vi "presentation_software.vi"() -> ()   [LabVIEW 2014]
uses:
  stateCtl.ctl
  <vilib>/Instr/_visa.llb/VISA Configure Serial Port (Instr).vi
panel:
  in  "AnalogOutputDT":dbl(slide) scale=0.0..100.0
  out "Led1":bool
  in  "Output1":bool
  out "Led0":bool
  in  "Output0":bool
  out "S6":dbl
  out "S5":dbl
  out "S4":dbl
  out "S3":dbl
  out "S2":dbl
  out "S1":dbl
  out "S0":dbl
  in  "Tab Control":T1(tab)
  out "Frequency":dbl(graph)
  out "Temperature 1":dbl(graph)
  out "Temperature 2":dbl(graph)
  out "Load Cell 1":dbl(graph)
  out "Load Cell 2":dbl(graph)
  out "Vibration":dbl(graph)
  out "Analog Output":dbl(graph)
  out "exitLed":bool
  out "statusBar":string="     "
  in  "startButton":bool
  out "stopLed":bool
  out "startLed":bool
  in  "VISA Serial Port":refnum<visa-resource-name>
  in  "exitButton":bool
  in  "stopButton":bool
  out "FE":string
  out "FP":string
  out "isRunning":bool
  out "state":T2=enum."exit"
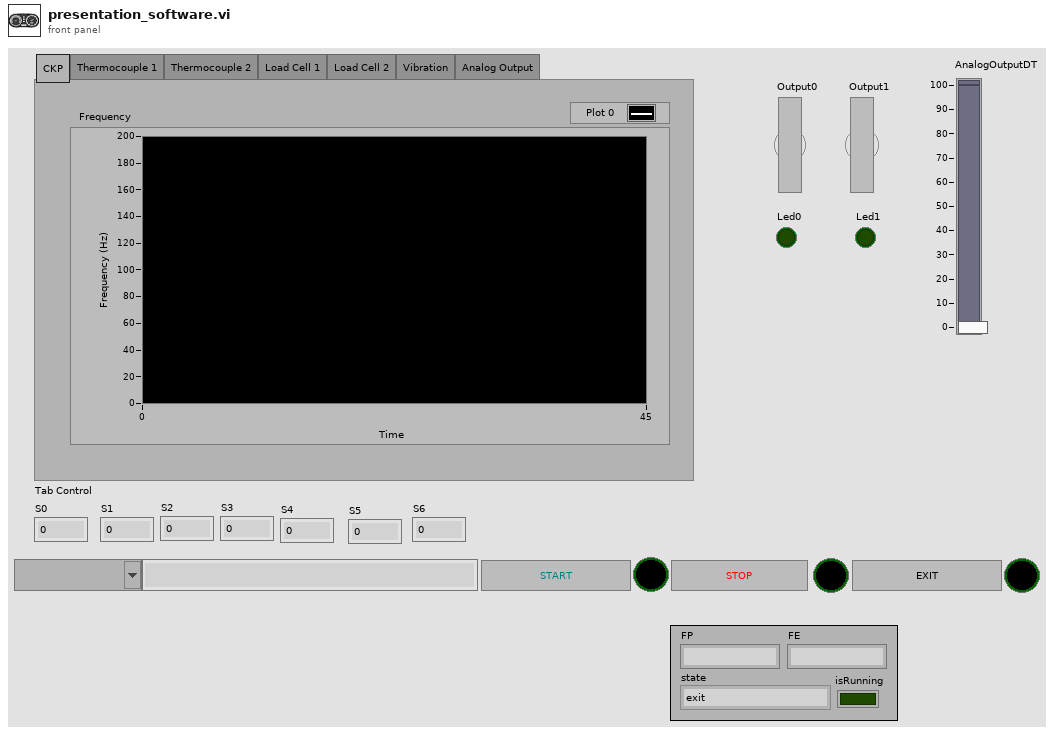
[diagram p1: front panel]
types:
  T1 = enum32{"CKP", "Thermocouple 1", "Thermocouple 2", "Load Cell 1", "Load Cell 2", "Vibration", "Analog Output"}
  T2 = typedef "stateCtl.ctl" = enum16{"init", "ready", "running", "stopped", "exit"}
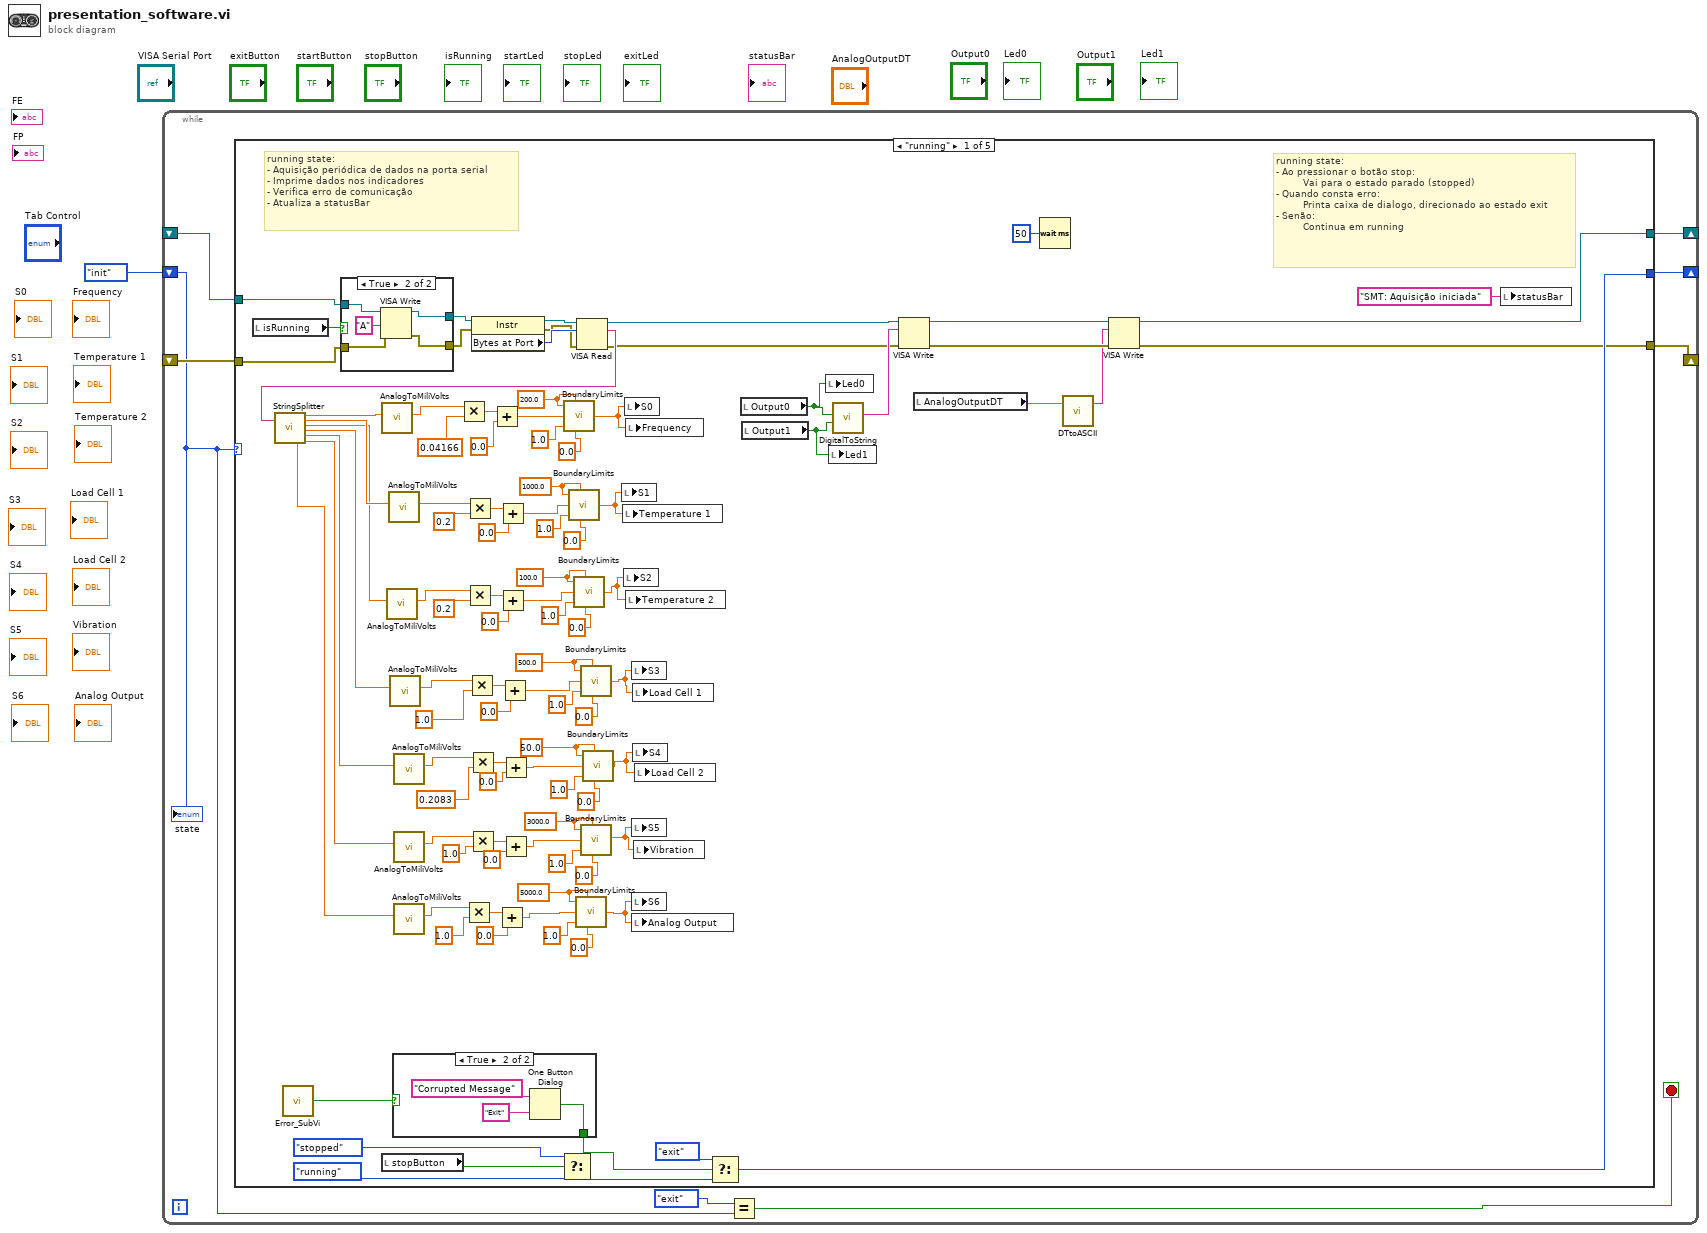
[diagram p0: block diagram]
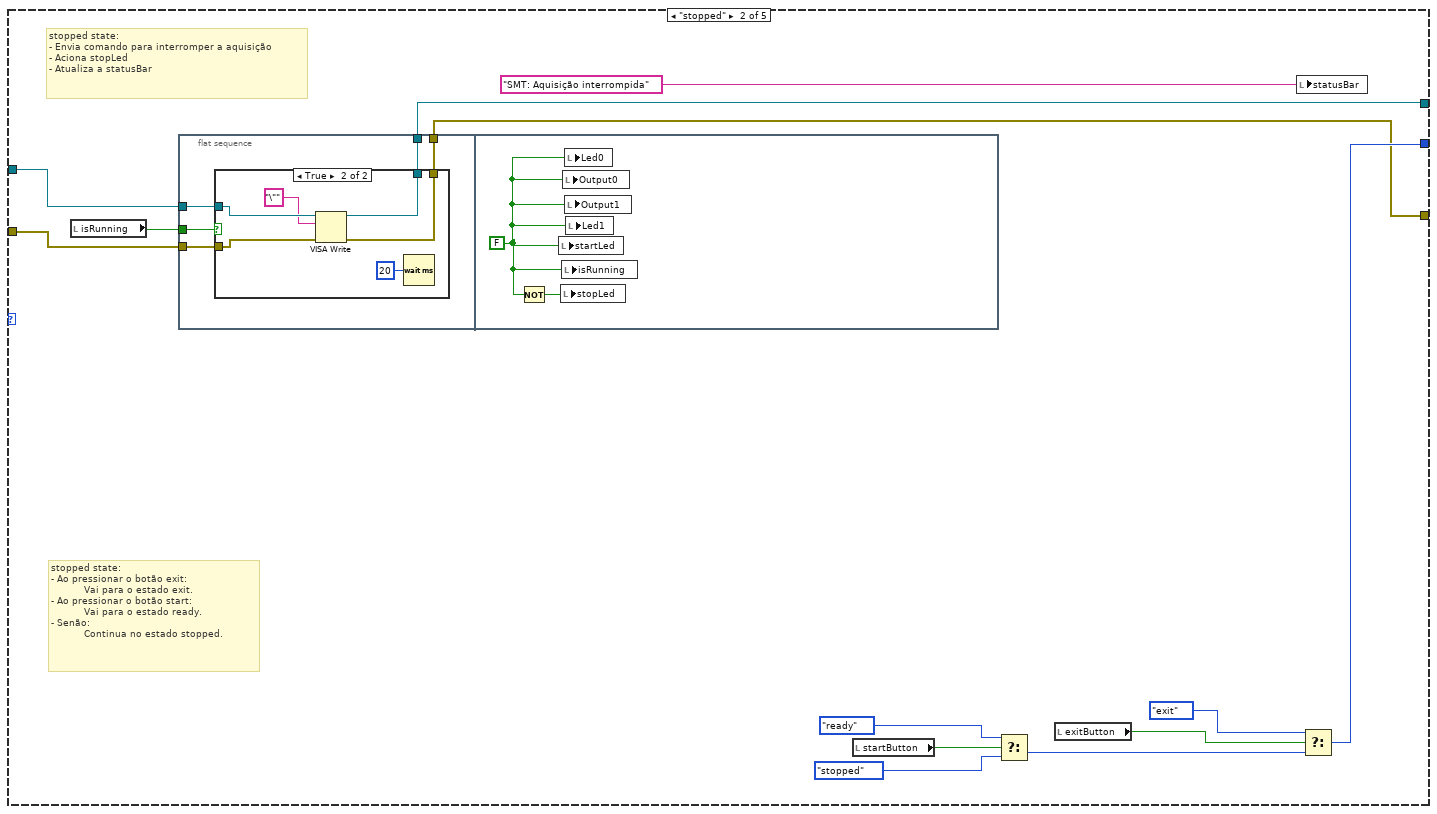
[diagram p4: hidden frame]
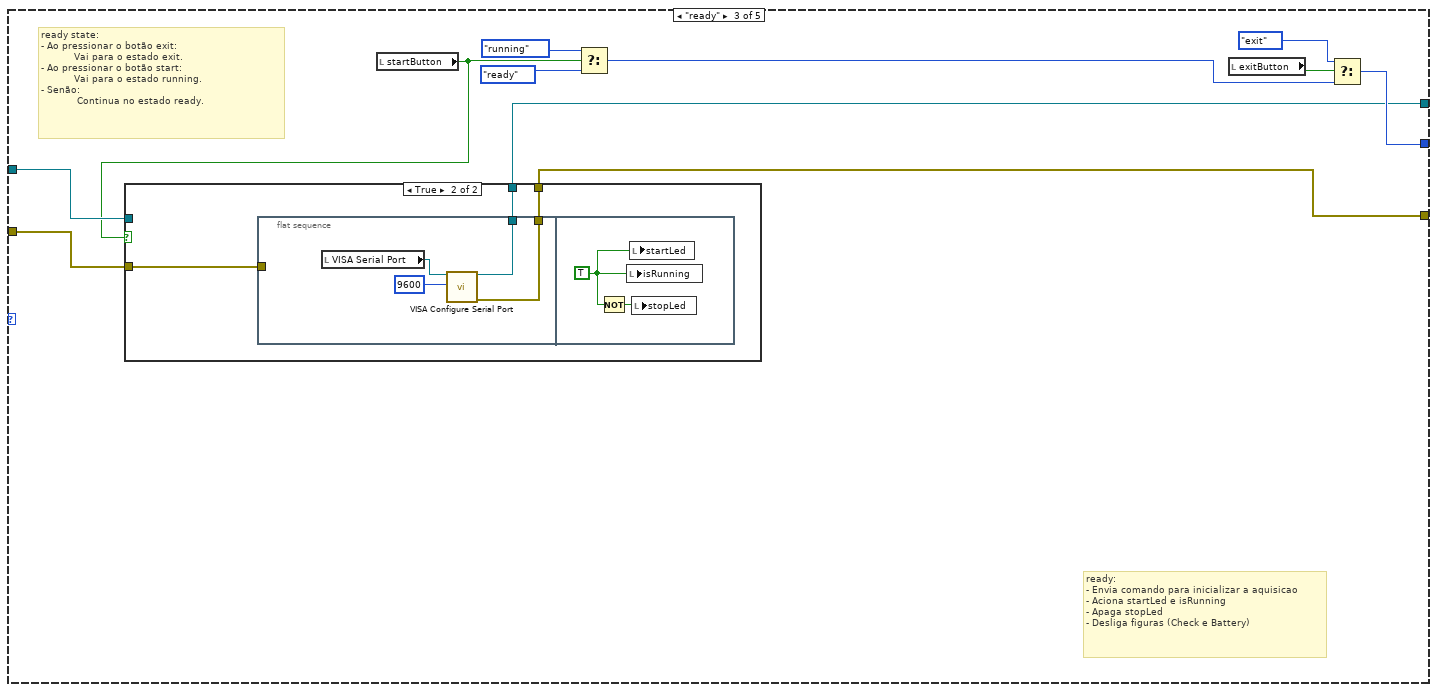
[diagram p6: hidden frame]
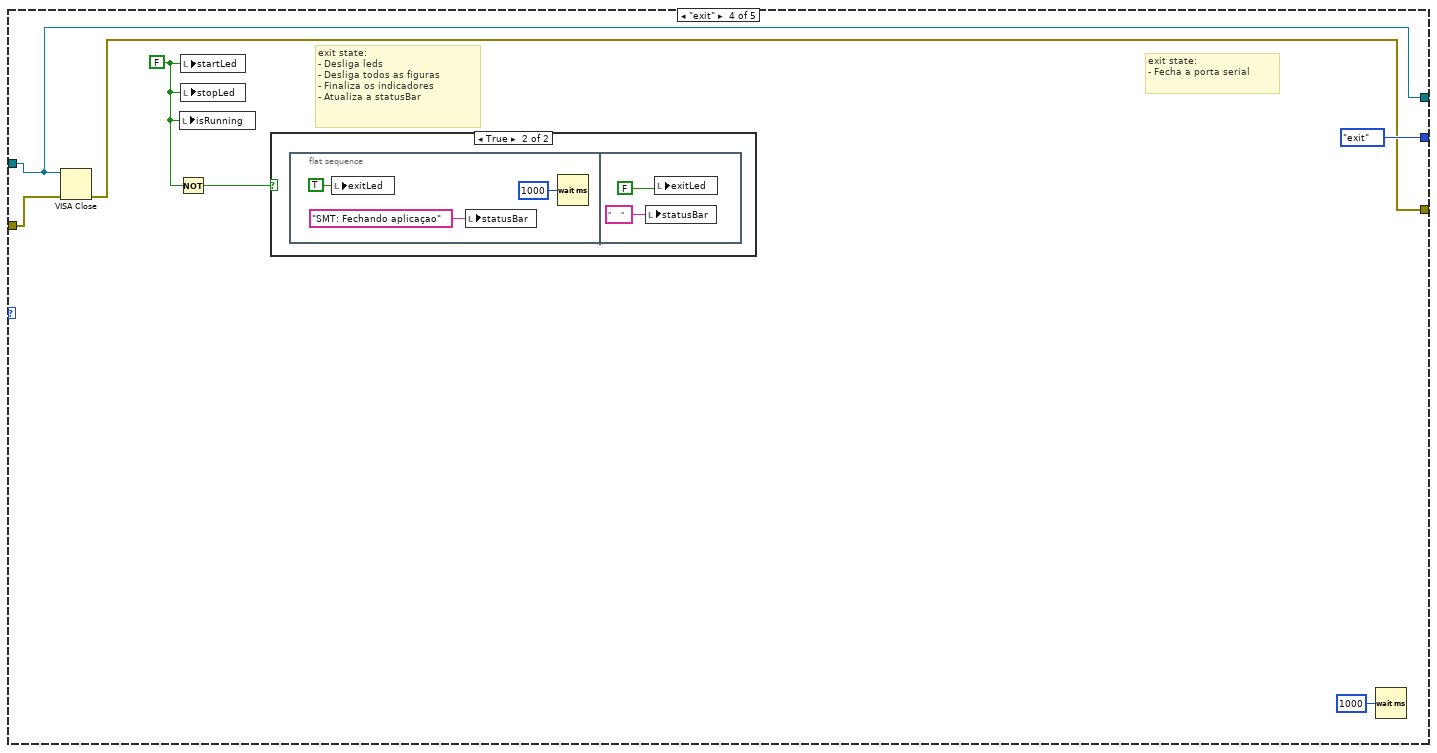
[diagram p8: hidden frame]
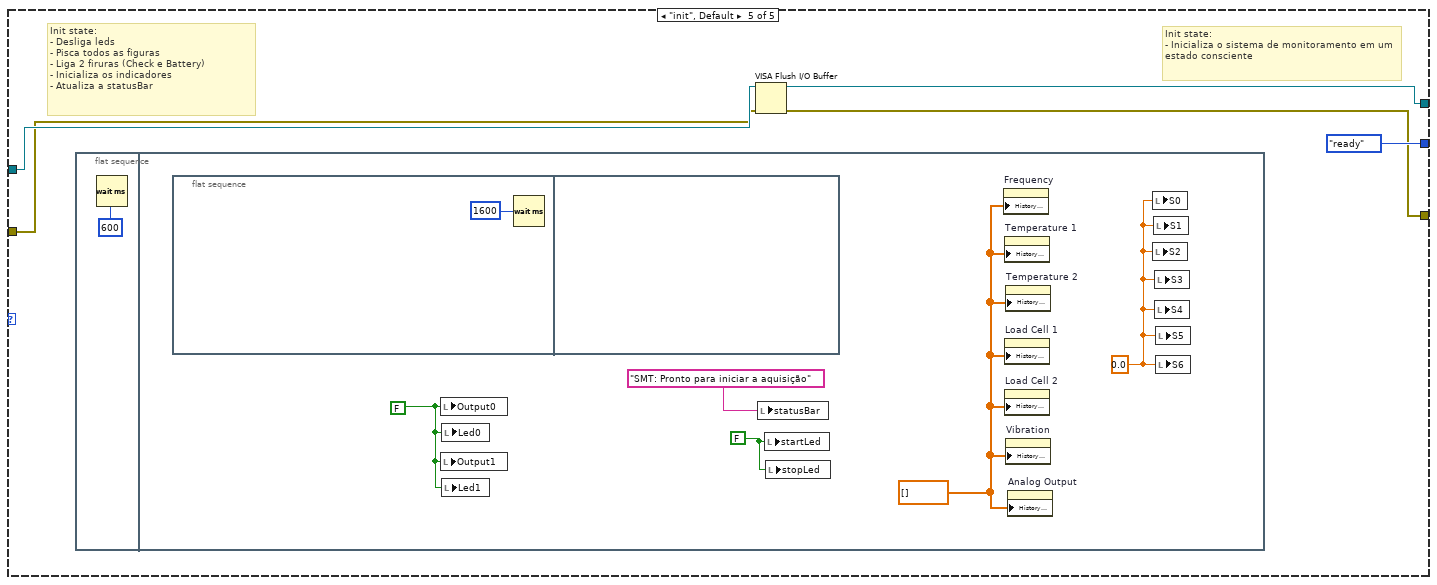
[diagram p10: hidden frame]
diagram:
  n1 = while {
    shift-right: [w3] -> _
    shift-left: _ -> [w8]
    shift-right: [w9] -> _
    shift-left: _ -> [w7]
    shift-right: [w4] -> _
    shift-left: stateCtl."init" ("state") -> [w5]
    stop <- w2 stop-if-true
    n2 = case shown="\"running\"" w5 {
      tunnel: [w11 w125 w151 w174 w184] -> w3
      tunnel: [w10 w126 w150 w175 w183] -> w9
      tunnel: [w103 w131 w154 stateCtl."exit" ("state") stateCtl."ready" ("state")] -> w4
      tunnel: w8 -> [w74 w129 w152 w174 w186]
      tunnel: w7 -> [w73 w128 w153 w176 w185]
      frame "running" {
        w36 = 5000.0
        w39 = 3000.0
        w42 = 50.0
        w47 = 500.0
        w52 = 100.0
        w57 = 1000.0
        w61 = 200.0
        # "running state:\n- Ao pressionar o botão stop: \n         Vai para o estado parado (stopped)\n- Quando consta erro:\n         Printa caixa de dialogo, direcionado ao estado exit  \n- Senão:          \n         Continua em running"
        # "running state:\n- Aquisição periódica de dados na porta serial\n- Imprime dados nos indicadores\n- Verifica erro de comunicação\n- Atualiza a statusBar"
        n3 = local read "isRunning"() -> (w100:bool)
        n4 = call "Error_SubVi.vi"() -> ("error"=w99:bool)  [unwired: 11 in]
        n5 = case shown="True" w100 {
          tunnel: [w115 w116] -> w71
          tunnel: [w114 w117] -> w72
          tunnel: w73 -> [w115 w119]
          tunnel: w74 -> [w114 w118]
          frame False {
          }
          frame True {
            n6 = VISA Write(VISA resource name=w118, write buffer="A", error in (no error)=w119) -> (VISA resource name out=w117:refnum<visa-resource-name>, error out=w116:errorcluster)  [unwired: 1 out]
          }
        }
        n7 = local read "stopButton"() -> (w107:bool)
        n8 = case shown="True" w99 {
          selector: w99 -> [w110 _]
          tunnel: [w110 w111] -> w101
          frame False {
          }
          frame True {
            n9 = One Button Dialog(message="Corrupted Message", button name ("OK")="Exit") -> (true=w111:bool)
          }
        }
        n10 = property class="Instr"(reference=w72, error in=w71) -> (reference out=w68:refnum<visa-resource-name>, error out=w69:errorcluster, "Bytes at Port"=w70:u32)
        n11 = Select(t=stateCtl."stopped" ("state"), s=w107, f=stateCtl."running" ("state")) -> (s? t:f=w102:T2)
        n12 = VISA Read(VISA resource name=w68, byte count=w70, error in (no error)=w69) -> (VISA resource name out=w17:refnum<visa-resource-name>, read buffer=w67:string, error out=w16:errorcluster)  [unwired: 1 out]
        n13 = call "StringSplitter.vi"("Input String"=w67) -> ("S6"=w75:dbl, "S0"=w81:dbl, "S1"=w80:dbl, "S2"=w79:dbl, "S3"=w78:dbl, "S4"=w77:dbl, "S5"=w76:dbl)  [unwired: 11 in, 1 out]
        n14 = call "AnalogToMiliVolts.vi"("Input"=w81) -> ("Output"=w82:dbl)  [unwired: 10 in]
        n15 = call "AnalogToMiliVolts.vi"("Input"=w79) -> ("Output"=w84:dbl)  [unwired: 10 in]
        n16 = call "AnalogToMiliVolts.vi"("Input"=w80) -> ("Output"=w83:dbl)  [unwired: 10 in]
        n17 = call "AnalogToMiliVolts.vi"("Input"=w78) -> ("Output"=w85:dbl)  [unwired: 10 in]
        n18 = call "AnalogToMiliVolts.vi"("Input"=w77) -> ("Output"=w86:dbl)  [unwired: 10 in]
        n19 = call "AnalogToMiliVolts.vi"("Input"=w76) -> ("Output"=w87:dbl)  [unwired: 10 in]
        n20 = call "AnalogToMiliVolts.vi"("Input"=w75) -> ("Output"=w88:dbl)  [unwired: 10 in]
        n21 = Multiply(x=w82, y=0.04166) -> (x*y=w97:dbl)
        n22 = Multiply(x=w88, y=1.0) -> (x*y=w89:dbl)
        n23 = Multiply(x=w83, y=0.2) -> (x*y=w95:dbl)
        n24 = Multiply(x=w84, y=0.2) -> (x*y=w93:dbl)
        n25 = Multiply(x=w85, y=1.0) -> (x*y=w92:dbl)
        n26 = Multiply(x=w86, y=0.2083) -> (x*y=w91:dbl)
        n27 = Multiply(x=w87, y=1.0) -> (x*y=w90:dbl)
        n28 = Add(x=w97, y=0.0) -> (x+y=w63:dbl)
        n29 = Add(x=w89, y=0.0) -> (x+y=w27:dbl)
        n30 = Add(x=w95, y=0.0) -> (x+y=w54:dbl)
        n31 = Add(x=w93, y=0.0) -> (x+y=w49:dbl)
        n32 = Add(x=w92, y=0.0) -> (x+y=w43:dbl)
        n33 = Add(x=w91, y=0.0) -> (x+y=w25:dbl)
        n34 = Add(x=w90, y=0.0) -> (x+y=w26:dbl)
        n35 = call "BoundaryLimits.vi"("UpperLimit"=w61, "UpperValue"=w61, "Input"=w63, "LowerLimit"=1.0, "LowerValue"=0.0) -> ("Output"=w62:dbl)
        n36 = call "BoundaryLimits.vi"("UpperLimit"=w57, "UpperValue"=w57, "Input"=w54, "LowerLimit"=1.0, "LowerValue"=0.0) -> ("Output"=w53:dbl)
        n37 = call "BoundaryLimits.vi"("UpperLimit"=w52, "UpperValue"=w52, "Input"=w49, "LowerLimit"=1.0, "LowerValue"=0.0) -> ("Output"=w48:dbl)
        n38 = call "BoundaryLimits.vi"("UpperLimit"=w36, "UpperValue"=w36, "Input"=w27, "LowerLimit"=1.0, "LowerValue"=0.0) -> ("Output"=w22:dbl)
        n39 = call "BoundaryLimits.vi"("UpperLimit"=w47, "UpperValue"=w47, "Input"=w43, "LowerLimit"=1.0, "LowerValue"=0.0) -> ("Output"=w44:dbl)
        n40 = call "BoundaryLimits.vi"("UpperLimit"=w39, "UpperValue"=w39, "Input"=w26, "LowerLimit"=1.0, "LowerValue"=0.0) -> ("Output"=w23:dbl)
        n41 = call "BoundaryLimits.vi"("UpperLimit"=w42, "UpperValue"=w42, "Input"=w25, "LowerLimit"=1.0, "LowerValue"=0.0) -> ("Output"=w24:dbl)
        n42 = local write "S1"(w53) -> ()
        n43 = local write "Temperature 1"(w53) -> ()
        n44 = local write "S2"(w48) -> ()
        n45 = local write "S0"(w62) -> ()
        n46 = local write "Frequency"(w62) -> ()
        n47 = local write "Temperature 2"(w48) -> ()
        n48 = local write "S3"(w44) -> ()
        n49 = local write "S5"(w23) -> ()
        n50 = local write "S6"(w22) -> ()
        n51 = local write "Analog Output"(w22) -> ()
        n52 = local write "Load Cell 1"(w44) -> ()
        n53 = local write "S4"(w24) -> ()
        n54 = local write "Vibration"(w23) -> ()
        n55 = local write "Load Cell 2"(w24) -> ()
        n56 = Select(t=stateCtl."exit" ("state"), s=w101, f=w102) -> (s? t:f=w103:T2)
        n57 = local read "Output0"() -> (w66:bool)
        n58 = local read "Output1"() -> (w65:bool)
        n59 = local write "Led0"(w66) -> ()
        n60 = local write "Led1"(w65) -> ()
        n61 = call "DigitalToString.vi"("D1"=w65, "D0"=w66) -> ("Out"=w64:string)  [unwired: 9 in]
        n62 = VISA Write(VISA resource name=w17, write buffer=w64, error in (no error)=w16) -> (VISA resource name out=w14:refnum<visa-resource-name>, error out=w13:errorcluster)  [unwired: 1 out]
        n63 = local read "AnalogOutputDT"() -> (w15:dbl)
        n64 = Wait (ms)(milliseconds to wait=u32 50) -> ()  [unwired: 1 out]
        n65 = call "DTtoASCII.vi"("Slide"=w15) -> ("ASCII"=w12:string)  [unwired: 1 in, 1 out]
        n66 = VISA Write(VISA resource name=w14, write buffer=w12, error in (no error)=w13) -> (VISA resource name out=w11:refnum<visa-resource-name>, error out=w10:errorcluster)  [unwired: 1 out]
        n67 = local write "statusBar"("SMT: Aquisição iniciada" ("statusBar")) -> ()
      }
      frame "stopped" {
        # "stopped state:\n- Ao pressionar o botão exit: \n           Vai para o estado exit.\n- Ao pressionar o botão start:\n           Vai para o estado ready.\n- Senão:\n           Continua no estado stopped."
        # "stopped state:\n- Envia comando para interromper a aquisição\n- Aciona stopLed\n- Atualiza a statusBar"
        n68 = local read "isRunning"() -> (w127:bool)
        n69 = flat-sequence {
          tunnel: w129 -> [w138]
          tunnel: w128 -> [w137]
          tunnel: w127 -> [w136]
          tunnel: [w135] -> w126
          tunnel: [w134] -> w125
          frame #0 {
            n70 = case shown="True" w136 {
              tunnel: w138 -> [w140 w146]
              tunnel: w137 -> [w139 w145]
              tunnel: [w139 w141] -> w135
              tunnel: [w140 w143] -> w134
              frame False {
              }
              frame True {
                n71 = VISA Write(VISA resource name=w146, write buffer="\"", error in (no error)=w145) -> (VISA resource name out=w143:refnum<visa-resource-name>, error out=w141:errorcluster)  [unwired: 1 out]
                n72 = Wait (ms)(milliseconds to wait=u32 20) -> ()  [unwired: 1 out]
              }
            }
          }
          frame #1 {
            w147 = FALSE ("Boolean")
            n73 = Not(x=w147) -> (.not. x?=w148:bool)
            n74 = local write "startLed"(w147) -> ()
            n75 = local write "stopLed"(w148) -> ()
            n76 = local write "isRunning"(w147) -> ()
            n77 = local write "Output0"(w147) -> ()
            n78 = local write "Led0"(w147) -> ()
            n79 = local write "Output1"(w147) -> ()
            n80 = local write "Led1"(w147) -> ()
          }
        }
        n81 = local read "startButton"() -> (w124:bool)
        n82 = Select(t=stateCtl."ready" ("state"), s=w124, f=stateCtl."stopped" ("state")) -> (s? t:f=w132:T2)
        n83 = local read "exitButton"() -> (w123:bool)
        n84 = local write "statusBar"("SMT: Aquisição interrompida" ("statusBar")) -> ()
        n85 = Select(t=stateCtl."exit" ("state"), s=w123, f=w132) -> (s? t:f=w131:T2)
      }
      frame "ready" {
        # "ready state:\n- Ao pressionar o botão exit: \n           Vai para o estado exit.\n- Ao pressionar o botão start:\n           Vai para o estado running.\n- Senão:\n            Continua no estado ready."
        # "ready:\n- Envia comando para inicializar a aquisicao\n- Aciona startLed e isRunning\n- Apaga stopLed\n- Desliga figuras (Check e Battery)"
        n86 = local read "startButton"() -> (w149:bool)
        n87 = case shown="True" w149 {
          tunnel: [w161 w162] -> w151
          tunnel: [w160 w163] -> w150
          tunnel: w152 -> [w161 _]
          tunnel: w153 -> [w160 w164]
          frame False {
          }
          frame True {
            n88 = flat-sequence {
              tunnel: w164 -> [_]
              tunnel: [w166] -> w163
              tunnel: [w165] -> w162
              frame #0 {
                n89 = local read "VISA Serial Port"() -> (w167:refnum<visa-resource-name>)
                n90 = call-poly "VISA Configure Serial Port"("VISA resource name"=w167, "baud rate (9600)"=u32 9600) -> ("VISA resource name out"=w165:refnum<visa-resource-name>, "error out"=w166:errorcluster)  [unwired: 12 in]
              }
              frame #1 {
                w170 = TRUE ("Boolean")
                n91 = Not(x=w170) -> (.not. x?=w169:bool)
                n92 = local write "isRunning"(w170) -> ()
                n93 = local write "startLed"(w170) -> ()
                n94 = local write "stopLed"(w169) -> ()
              }
            }
          }
        }
        n95 = Select(t=stateCtl."running" ("state"), s=w149, f=stateCtl."ready" ("state")) -> (s? t:f=w155:T2)
        n96 = local read "exitButton"() -> (w157:bool)
        n97 = Select(t=stateCtl."exit" ("state"), s=w157, f=w155) -> (s? t:f=w154:T2)
      }
      frame "exit" {
        w172 = FALSE ("startLed")
        # "exit state:\n- Desliga leds\n- Desliga todos as figuras\n- Finaliza os indicadores\n- Atualiza a statusBar"
        # "exit state:\n- Fecha a porta serial"
        n98 = VISA Close(VISA resource name=w174, error in (no error)=w176) -> (error out=w175:errorcluster)
        n99 = Not(x=w172) -> (.not. x?=w173:bool)
        n100 = local write "isRunning"(w172) -> ()
        n101 = local write "startLed"(w172) -> ()
        n102 = local write "stopLed"(w172) -> ()
        n103 = case shown="True" w173 {
          frame False {
          }
          frame True {
            n104 = flat-sequence {
              frame #0 {
                n105 = local write "exitLed"(TRUE ("exitLed")) -> ()
                n106 = local write "statusBar"("SMT: Fechando aplicaçao" ("statusBar")) -> ()
                n107 = Wait (ms)(milliseconds to wait=u32 1000) -> ()  [unwired: 1 out]
              }
              frame #1 {
                n108 = local write "statusBar"("     " ("statusBar")) -> ()
                n109 = local write "exitLed"(FALSE ("exitLed")) -> ()
              }
            }
          }
        }
        n110 = Wait (ms)(milliseconds to wait=u32 1000) -> ()  [unwired: 1 out]
      }
      frame "init", Default {
        # "Init state:\n- Inicializa o sistema de monitoramento em um estado consciente"
        # "Init state:\n- Desliga leds\n- Pisca todos as figuras\n- Liga 2 firuras (Check e Battery)\n- Inicializa os indicadores\n- Atualiza a statusBar"
        n111 = flat-sequence {
          frame #0 {
            n112 = Wait (ms)(milliseconds to wait=u32 600) -> ()  [unwired: 1 out]
          }
          frame #1 {
            w189 = dbl[] [] ("History Data")
            w190 = 0.0
            w191 = FALSE
            w193 = FALSE
            n113 = flat-sequence {
              frame #0 {
                n114 = Wait (ms)(milliseconds to wait=u32 1600) -> ()  [unwired: 1 out]
              }
              frame #1 {
              }
            }
            n115 = local write "Output0"(w191) -> ()
            n116 = local write "Output1"(w191) -> ()
            n117 = local write "Led0"(w191) -> ()
            n118 = local write "Led1"(w191) -> ()
            n119 = local write "statusBar"("SMT: Pronto para iniciar a aquisição" ("statusBar")) -> ()
            n120 = local write "startLed"(w193) -> ()
            n121 = local write "stopLed"(w193) -> ()
            n122 = property on="Frequency" class="WFChart (strict)"("History Data"=w189) -> ()  [unwired: 2 in, 2 out]
            n123 = property on="Temperature 1" class="WFChart (strict)"("History Data"=w189) -> ()  [unwired: 2 in, 2 out]
            n124 = property on="Load Cell 1" class="WFChart (strict)"("History Data"=w189) -> ()  [unwired: 2 in, 2 out]
            n125 = property on="Load Cell 2" class="WFChart (strict)"("History Data"=w189) -> ()  [unwired: 2 in, 2 out]
            n126 = property on="Temperature 2" class="WFChart (strict)"("History Data"=w189) -> ()  [unwired: 2 in, 2 out]
            n127 = property on="Vibration" class="WFChart (strict)"("History Data"=w189) -> ()  [unwired: 2 in, 2 out]
            n128 = property on="Analog Output" class="WFChart (strict)"("History Data"=w189) -> ()  [unwired: 2 in, 2 out]
            n129 = local write "S0"(w190) -> ()
            n130 = local write "S2"(w190) -> ()
            n131 = local write "S1"(w190) -> ()
            n132 = local write "S3"(w190) -> ()
            n133 = local write "S4"(w190) -> ()
            n134 = local write "S5"(w190) -> ()
            n135 = local write "S6"(w190) -> ()
          }
        }
        n136 = VISA Flush I/O Buffer(VISA resource name=w186, error in (no error)=w185) -> (VISA resource name out=w184:refnum<visa-resource-name>, error out=w183:errorcluster)  [unwired: 1 in]
      }
    }
    n137 = Equal?(x=stateCtl."exit" ("state"), y=w5) -> (x = y?=w2:bool)
    "state" <- w5
  }
